vi "frames_to_waveforms.vi"(0 "bg frames":dbl[][](array[numeric]), 1 "dt":dbl, 2 "mol frames":dbl[][](array[numeric])) -> (4 "bg waves":waveform(dbl)[](array[waveform]), 6 "mol waves":waveform(dbl)[](array[waveform]))   [LabVIEW 2011]
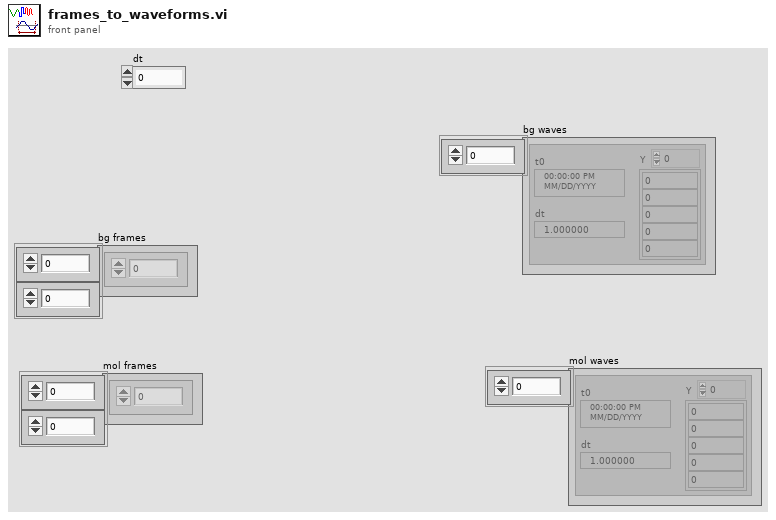
[diagram p1: front panel]
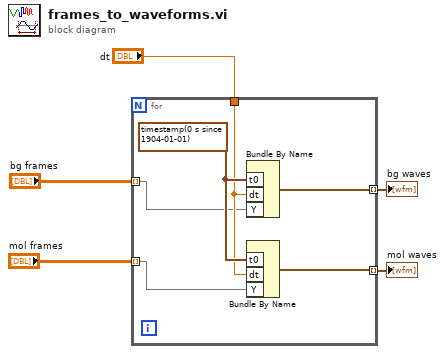
[diagram p0: block diagram]
diagram:
  n1 = for {
    tunnel: "bg frames" -> [w9] mode=indexing
    tunnel: "dt" -> [w10]
    tunnel: "mol frames" -> [w7] mode=indexing
    tunnel: [w8] -> w2 mode=indexing
    tunnel: [w6] -> w1 mode=indexing
    w11 = timestamp(0 s since 1904-01-01) ("t0")
    n2 = Bundle By Name("t0"=w11, "dt"=w10, "Y"=w9) -> (w8:waveform(dbl))  [unwired: 1 in]
    n3 = Bundle By Name("t0"=w11, "dt"=w10, "Y"=w7) -> (w6:waveform(dbl))  [unwired: 1 in]
  }
  "bg waves" <- w2
  "mol waves" <- w1
